vi "EDGE DETECTION REPORT.vi"(8 "error in (no error)":errorcluster, 9 "return value 2":cluster{string, string, dbl, dbl, dbl}, 10 "return value":cluster{string, dbl, dbl, dbl}, 11 "Main Ref":T1) -> (0 "error out":errorcluster)   [LabVIEW 2025]
uses:
  <vilib>/Exaprom PDF/Controls/Font Controls/Font complete cluster.ctl
  <vilib>/Exaprom PDF/Controls/Font Controls/Font size.ctl
  <vilib>/Exaprom PDF/Controls/Font Controls/Font color.ctl
  <vilib>/Exaprom PDF/Controls/Font Controls/Type and encoding.ctl
  <vilib>/Exaprom PDF/Controls/Text Controls/Unicode/Type and run direction.ctl
  <vilib>/Exaprom PDF/Controls/Header, Footer and Watermark Controls/Header or Footer  Text cluster.ctl
  <vilib>/Exaprom PDF/Controls/Table Controls/Cell Alignment 20px.ctl
  <vilib>/Exaprom PDF/Controls/Text Controls/Line spacing.ctl
  <vilib>/Exaprom PDF/Controls/Font Controls/Font complete cluster horizontal.ctl
  <vilib>/Exaprom PDF/Controls/Header, Footer and Watermark Controls/Header or Footer Line cluster.ctl
  <vilib>/Exaprom PDF/Controls/Header, Footer and Watermark Controls/Header Footer Line.ctl
  <vilib>/Exaprom PDF/Controls/Header, Footer and Watermark Controls/Watermark Text Cluster.ctl
  <vilib>/Exaprom PDF/Controls/Header, Footer and Watermark Controls/Watermark Position.ctl
  <vilib>/Exaprom PDF/Controls/Header, Footer and Watermark Controls/Header footer horiz alignment.ctl
  <vilib>/Exaprom PDF/Controls/Table Controls/Table properties.ctl
  <vilib>/Exaprom PDF/Controls/Table Controls/Table position.ctl
  <vilib>/Exaprom PDF/Controls/Header, Footer and Watermark Controls/Header or Footer.ctl
  <vilib>/Exaprom PDF/Controls/Image Controls/Image border.ctl
  <vilib>/Exaprom PDF/Controls/Header, Footer and Watermark Controls/Header or Footer  Image cluster.ctl
  <vilib>/Exaprom PDF/Controls/Table Controls/Cell Font, type, Alignment and LS V2.ctl
  <vilib>/Exaprom PDF/Controls/Table Controls/Cell Type, Alignment and LS.ctl
  <vilib>/Exaprom PDF/Controls/Table Controls/Text vertical arrangement.ctl
  <vilib>/Exaprom PDF/Controls/Image Controls/Image alignment and position.ctl
  <vilib>/Exaprom PDF/Controls/Image Controls/Image aligment.ctl
  <vilib>/Exaprom PDF/VIs/Low level/Header, Footer and Watermark Low level/Append Image HF.vi
  <vilib>/Exaprom PDF/VIs/Low level/Header, Footer and Watermark Low level/Append Text HF.vi
  <vilib>/Exaprom PDF/VIs/Low level/Header, Footer and Watermark Low level/AppendLine seperator.vi
  <vilib>/Exaprom PDF/VIs/Text/Append Phrase.vi
  <vilib>/Exaprom PDF/VIs/Low level/Header, Footer and Watermark Low level/Append Watermark Text.vi
panel:
  in  "Watermark Text 2":T2={"Text "="PALTRO", "Opacity (%)"=5.0, "Position"={"Position"=enum."Center (text section)", "X"=0.0, "Y"=0.0}, "Automatic"=TRUE, "Font"={"Font Name"="", "Size"=-1.0, "Color"=0}, "Alignment"=enum."Center", "Rotate(°)"=0.0}
  in  "Footer Line 2":T7={"H/F Line"=enum."Horizontal line", "Thickness (point)"=0.75, " Colour"=7171459}
  in  "Header Line":T7={"H/F Line"=enum."Horizontal line", "Thickness (point)"=0.75, " Colour"=7171459}
  in  "Footer Text":T9={"Start at page"=1, "Cell Alignment"=4, "Line spacing"=enum."Select", "Text"="Fully automated next-gen fuel and lubricant testers: BOCLE 2.0 , HFRR adv , FBT 3.0", "Font complete"={"Name"="", "Size"=6.0, "Color"=16777224, "Style"={"Bold"=FALSE, "Italic"=FALSE, "Underline"=TRUE, "Strikeout"=FALSE}, "Type"={"Type&direction"=enum."Select", "Embedded"=FALSE, "Encoding"=""}}, "Link"="https://www.paltro.com/products/product-selector/lubricity"}
  in  "Date and Time :":string
  in  "Observations :":string
  in  "Scar Image Path :":path
  in  "Header or footer":T9={"Start at page"=1, "Cell Alignment"=4, "Line spacing"=enum."Select", "Text"="                                            ", "Font complete"={"Name"="", "Size"=-1.0, "Color"=0, "Style"={"Bold"=FALSE, "Italic"=FALSE, "Underline"=FALSE, "Strikeout"=FALSE}, "Type"={"Type&direction"=enum."Select", "Embedded"=FALSE, "Encoding"=""}}, "Link"=""}
  in  "Font":T15={"Name"="", "Size"=18.0, "Color"=0, "Style"={"Bold"=TRUE, "Italic"=FALSE, "Underline"=FALSE, "Strikeout"=FALSE}, "Type"={"Type&direction"=enum."Select", "Embedded"=FALSE, "Encoding"=""}}
  in  "Font 2":T15={"Name"="", "Size"=6.0, "Color"=0, "Style"={"Bold"=FALSE, "Italic"=TRUE, "Underline"=FALSE, "Strikeout"=FALSE}, "Type"={"Type&direction"=enum."Select", "Embedded"=FALSE, "Encoding"=""}}
  in  "File Name :":string(combo)
  out "folder names":string[](array[string])
  out "path out":path
  in  "Automated":bool
  in  "Test Method":string
  in  "Fuel Description":string
  out "Operator :":string
types:
  T1 = cluster{"File Name":string, "Test Method":string, "Operator":string, "Fuel Description":string, "Date and time":string}
  T2 = typedef "Watermark Text Cluster.ctl" = cluster{"Text ":string, "Opacity (%)":sgl, "Position":cluster{"Position":T3, "X":sgl, "Y":sgl}, "Automatic":bool, "Font":cluster{"Font Name":string, "Size":T4, "Color":T5}, "Alignment":T6, "Rotate(°)":sgl}
  T3 = typedef "Watermark Position.ctl" = enum16{"Absolute", "Center (page)", "Center (text section)"}
  T4 = typedef "Font size.ctl" = sgl
  T5 = typedef "Font color.ctl" = u32
  T6 = typedef "Header footer horiz alignment.ctl" = enum16{"Left", "Center", "Right"}
  T7 = typedef "Header or Footer Line cluster.ctl" = cluster{"H/F Line":T8, "Thickness (point)":sgl, " Colour":u32}
  T8 = typedef "Header Footer Line.ctl" = enum16{"No line", "Horizontal line"}
  T9 = typedef "Header or Footer  Text cluster.ctl" = cluster{"Start at page":i32, "Cell Alignment":T10, "Line spacing":T11, "Text":string, "Font complete":T12, "Link":string}
  T10 = typedef "Cell Alignment 20px.ctl" = u16
  T11 = typedef "Line spacing.ctl" = enum16{"Select", "1.0", "1.5", "2.0"}
  T12 = typedef "Font complete cluster horizontal.ctl" = cluster{"Name":string, "Size":T4, "Color":T5, "Style":cluster{"Bold":bool, "Italic":bool, "Underline":bool, "Strikeout":bool}, "Type":T13}
  T13 = typedef "Type and encoding.ctl" = cluster{"Type&direction":T14, "Embedded":bool, "Encoding":string}
  T14 = typedef "Type and run direction.ctl" = enum16{"Select", "ASCII", "UTF-16", "UTF-16 (default)", "UTF-16 (LTR)", "UTF-16 (RTL)"}
  T15 = typedef "Font complete cluster.ctl" = cluster{"Name":string, "Size":T4, "Color":T5, "Style":cluster{"Bold":bool, "Italic":bool, "Underline":bool, "Strikeout":bool}, "Type":T13}
  T16 = typedef "Image alignment and position.ctl" = cluster{"Alignment":T17, "X ":sgl, "Y":sgl, "Indentation":sgl}
  T17 = typedef "Image aligment.ctl" = enum16{"Absolute (X,Y)", "Left", "Center", "Right", "Left (textwrap)", "Right (textwrap)"}
  T18 = typedef "Image border.ctl" = cluster{"Show?":bool, "Thickness (point)":sgl, "Color":u32}
  T19 = typedef "Cell Font, type, Alignment and LS V2.ctl" = cluster{"Cell Type, Alignment and LS":T20, "Font":T15}
  T20 = typedef "Cell Type, Alignment and LS.ctl" = cluster{"Cell Alignment":T10, "Text rotation":T21, "Line spacing":T11}
  T21 = typedef "Text vertical arrangement.ctl" = enum16{"None", "Clockwise", "Counterclockwise"}
  T22 = typedef "Header or Footer  Image cluster.ctl" = cluster{"Start at page":i32, "Cell Alignment":T10, "Path":path, "Image (%)":sgl, "Link":string}
  T23 = typedef "Table properties.ctl" = cluster{"Table position":T24, "SpacingBefore (points)":sgl, "SpacingAfter (points)":sgl}
  T24 = typedef "Table position.ctl" = i32
  T25 = typedef "Header or Footer.ctl" = enum16{"Header", "Footer"}
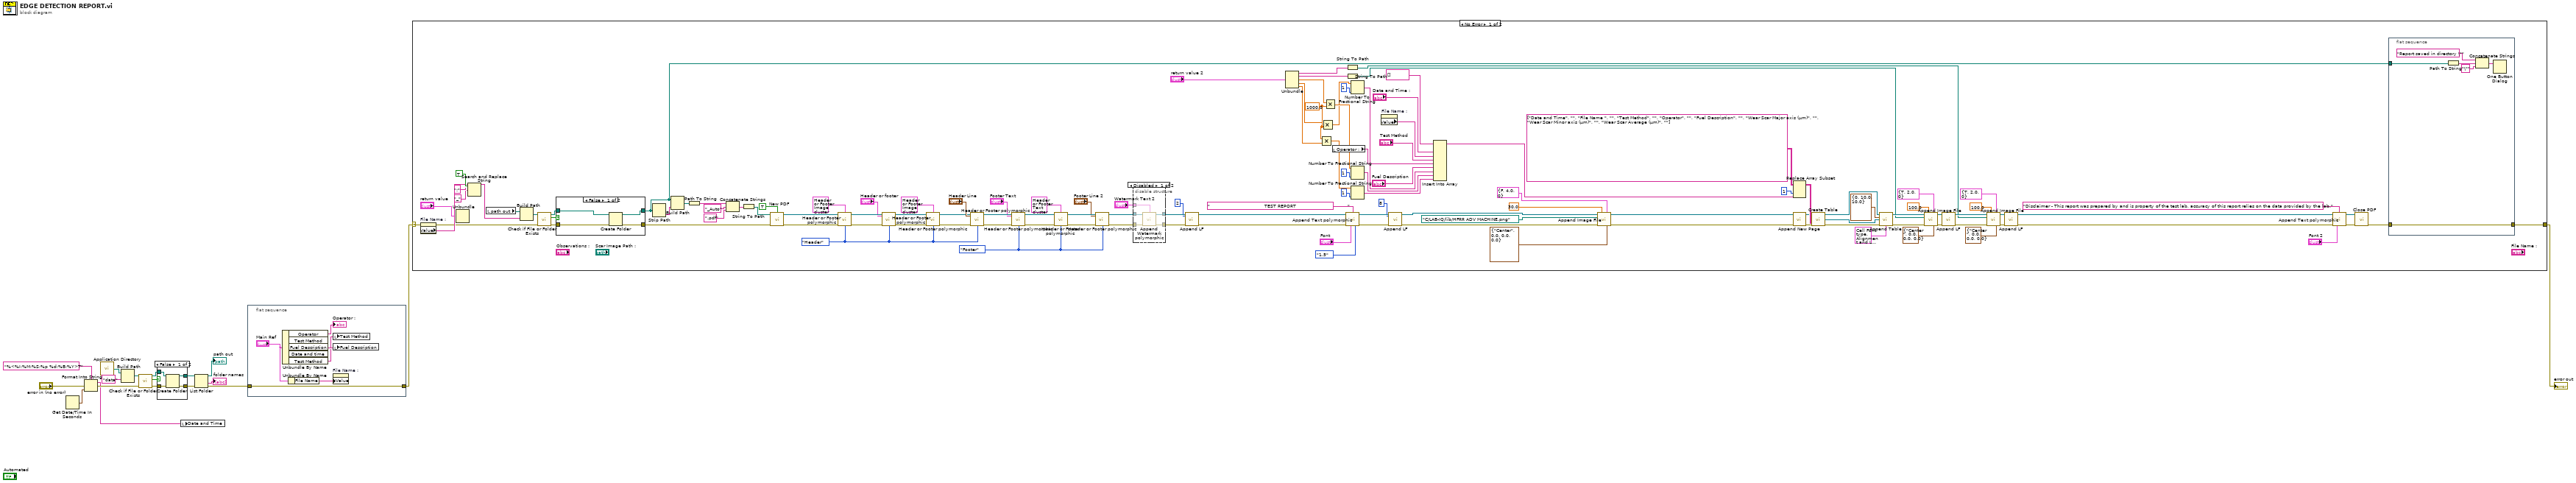
[diagram p0: block diagram]
diagram:
  n1 = Get Date/Time In Seconds() -> (seconds since 1Jan1904=w7:timestamp)
  n2 = Format Into String(format string="%<%I:%M:%S:%p %d:%B:%Y>T", error in="error in (no error)", w7) -> (resulting string=w1:string, error out=w5:errorcluster)  [unwired: 1 in]
  n3 = call <vilib>:"Application Directory.vi"() -> ("Application Directory"=w9:path)
  n4 = Build Path(base path=w9, name or relative path="data") -> (appended path=w8:path)
  n5 = call <vilib>:"Check if File or Folder Exists.vi"("error in (no error)"=w5, "path"=w8) -> ("error out"=w13:errorcluster, "file or folder exists?"=w15:bool, "dup path"=w14:path)  [unwired: 7 in]
  n6 = case shown="False" w15 {
    tunnel: w14 -> [w22 w23]
    tunnel: w13 -> [w21 w24]
    tunnel: [w20 w24] -> w18
    tunnel: [w19 w23] -> w16
    frame False {
      n7 = Create Folder(path (use dialog)=w22, error in=w21) -> (created path=w19:path, error out=w20:errorcluster)  [unwired: 1 in, 1 out]
    }
    frame True {
    }
  }
  n8 = local write "Date and Time :"(w1) -> ()
  n9 = List Folder(path=w16, error in=w18) -> (path out=→"path out":path, folder names=→"folder names":string[], error out=w3:errorcluster)  [unwired: 2 in, 1 out]
  n10 = flat-sequence {
    tunnel: w3 -> [w26]
    tunnel: [w26] -> w2
    frame #0 {
      n11 = Unbundle By Name("Main Ref") -> ("Operator"=→"Operator :":string, "Fuel Description"=w27:string, "Test Method"=w25:string)  [unwired: 2 out]
      n12 = Unbundle By Name("Main Ref") -> ("File Name"=w30:string)
      n13 = local write "Test Method"(w25) -> ()
      n14 = local write "Fuel Description"(w27) -> ()
      n15 = property on="File Name :" class="CmbBox"("Value"=w30) -> ()  [unwired: 2 in, 2 out]
    }
  }
  n16 = case shown="No Error" w2 {
    selector: w2 -> [w64 _]
    tunnel: [w59 _] -> w11
    frame No Error {
      w38 = 1000.0 ("y")
      w79 = Header_or_Footer."Header" ("Position")
      w109 = Header_or_Footer."Footer" ("Position")
      n17 = property on="File Name :" class="CmbBox"(error in=w64) -> (error out=w68:errorcluster, "Value"=w69:string)  [unwired: 1 in, 1 out]
      n18 = Unbundle("return value") -> ()  [unwired: 4 out]
      n19 = Search and Replace String(replace all?=TRUE ("replace all? (F)"), input string=w69, search string=":", replace string="_" ("replace string (\"\")")) -> (result string=w99:string)  [unwired: 4 in, 3 out]
      n20 = local read "path out"() -> (w70:path)
      n21 = Build Path(base path=w70, name or relative path=w99) -> (appended path=w126:path)
      n22 = call <vilib>:"Check if File or Folder Exists.vi"("error in (no error)"=w68, "path"=w126) -> ("error out"=w123:errorcluster, "file or folder exists?"=w125:bool, "dup path"=w124:path)  [unwired: 7 in]
      n23 = case shown="False" w125 {
        tunnel: w124 -> [w172 w173]
        tunnel: w123 -> [w171 w174]
        tunnel: [w170 w174] -> w122
        tunnel: [w169 w173] -> w71
        frame False {
          n24 = Create Folder(path (use dialog)=w172, error in=w171) -> (created path=w169:path, error out=w170:errorcluster)  [unwired: 1 in, 1 out]
        }
        frame True {
        }
      }
      n25 = Strip Path(path=w71) -> (name=w128:string)  [unwired: 1 out]
      n26 = Build Path(base path=w71, name or relative path=w128) -> (appended path=w127:path)
      n27 = Path To String(path=w127) -> (string=w58:string)
      n28 = Concatenate Strings(w58, "_Auto" ("string"), ".pdf" ("string")) -> (w129:string)
      n29 = String To Path(string=w129) -> (path=w121:path)
      n30 = call <vilib>:"New PDF.vi"("PDF Path"=w121, "Overwrite?"=TRUE, "error in (no error)"=w122) -> ("PDF Report"=w143:refnum<class "PDF Report Class.lvclass">, "error out"=w144:errorcluster)  [unwired: 11 in]
      n31 = call-poly <vilib>:"Header or Footer polymorphic.vi"("PDF Report IN"=w143, "Header or footer"=T22 {"Start at page"=1, "Cell Alignment"=4, "Path"=path "C:/LAB-IQ/lib/paltro logo.png", "Image (%)"=100.0, "Link"="https://www.paltro.com/"} ("HEADER Image"), "error in (no error)"=w144, "Position"=w79) -> ("PDF Report OUT"=w97:refnum<class "PDF Report Class.lvclass">, "error out"=w98:errorcluster)  [unwired: 10 out]
      n32 = call-poly <vilib>:"Header or Footer polymorphic.vi"("PDF Report IN"=w97, "Header or footer"="Header or footer", "error in (no error)"=w98, "Position"=w79) -> ("PDF Report OUT"=w95:refnum<class "PDF Report Class.lvclass">, "error out"=w96:errorcluster)  [unwired: 10 out]
      n33 = call-poly <vilib>:"Header or Footer polymorphic.vi"("PDF Report IN"=w95, "Header or footer"=T22 {"Start at page"=1, "Cell Alignment"=6, "Path"=path "C:/LAB-IQ/lib/HFRR_adv.png", "Image (%)"=30.0, "Link"="https://www.paltro.com/products/test-and-measurement/bocle--automated-ball-on-cylinder-lubricity-evaluator"} ("HEADER Image  2"), "error in (no error)"=w96, "Position"=w79) -> ("PDF Report OUT"=w115:refnum<class "PDF Report Class.lvclass">, "error out"=w116:errorcluster)  [unwired: 10 out]
      n34 = call-poly <vilib>:"Header or Footer polymorphic.vi"("PDF Report IN"=w115, "H/F Line"="Header Line", "error in (no error)"=w116, "Position"=w79) -> ("PDF Report OUT"=w147:refnum<class "PDF Report Class.lvclass">, "error out"=w146:errorcluster)  [unwired: 1 in, 9 out]
      n35 = call-poly <vilib>:"Header or Footer polymorphic.vi"("PDF Report IN"=w147, "Header or footer"="Footer Text", "error in (no error)"=w146, "Position"=w109) -> ("PDF Report OUT"=w149:refnum<class "PDF Report Class.lvclass">, "error out"=w148:errorcluster)  [unwired: 10 out]
      n36 = call-poly <vilib>:"Header or Footer polymorphic.vi"("PDF Report IN"=w149, "Header or footer"=T9 {"Start at page"=1, "Cell Alignment"=6, "Line spacing"=enum."Select", "Text"="www.paltro.com", "Font complete"={"Name"="", "Size"=6.0, "Color"=16777224, "Style"={"Bold"=FALSE, "Italic"=FALSE, "Underline"=TRUE, "Strikeout"=FALSE}, "Type"={"Type&direction"=enum."Select", "Embedded"=FALSE, "Encoding"=""}}, "Link"="https://www.paltro.com/"} ("Footer Text 2"), "error in (no error)"=w148, "Position"=w109) -> ("PDF Report OUT"=w142:refnum<class "PDF Report Class.lvclass">, "error out"=w141:errorcluster)  [unwired: 10 out]
      n37 = call-poly <vilib>:"Header or Footer polymorphic.vi"("PDF Report IN"=w142, "H/F Line"="Footer Line 2", "error in (no error)"=w141, "Position"=w109) -> ("PDF Report OUT"=w135:refnum<class "PDF Report Class.lvclass">, "error out"=w136:errorcluster)  [unwired: 1 in, 9 out]
      n38 = disable-structure shown="Disabled" {
        disable-tunnel: "Watermark Text 2" -> [w166 _]
        disable-tunnel: w136 -> [w165 w168]
        disable-tunnel: w135 -> [w164 w167]
        disable-tunnel: [w163 w168] -> w91
        disable-tunnel: [w162 w167] -> w90
        frame Disabled {
          n39 = call-poly <vilib>:"Append Watermark polymorphic.vi"("PDF Report IN"=w164, "Watermark Text"=w166, "error in (no error)"=w165) -> ("PDF Report OUT"=w162:refnum<class "PDF Report Class.lvclass">, "error out"=w163:errorcluster)  [unwired: 1 in, 10 out]
        }
        frame Enabled {
        }
      }
      n40 = call <vilib>:"Append LF.vi"("PDF Report IN"=w90, "Number of LF (default 1)"=u8 2, "error in (no error)"=w91) -> ("PDF Report duplicate"=w88:refnum<class "PDF Report Class.lvclass">, "error out"=w89:errorcluster)  [unwired: 11 in]
      n41 = Unbundle("return value 2") -> (w44:string, w45:string, w37:dbl, w36:dbl, w35:dbl)
      n42 = Multiply(x=w38, y=w35) -> (x*y=w32:dbl)
      n43 = Multiply(x=w36, y=w38) -> (x*y=w33:dbl)
      n44 = Multiply(x=w37, y=w38) -> (x*y=w34:dbl)
      n45 = local read "Operator :"() -> (w31:string)
      n46 = String To Path(string=w44) -> (path=w42:path)
      n47 = String To Path(string=w45) -> (path=w43:path)
      n48 = call-poly <vilib>:"Append Text polymorphic.vi"("PDF Report IN"=w88, "Text"="                                     TEST REPORT                                   ", "error in (no error)"=w89, "Font"="Font", "Line spacing"=Line_spacing."1.5") -> ("PDF Report OUT"=w75:refnum<class "PDF Report Class.lvclass">, "error out"=w76:errorcluster)  [unwired: 9 in]
      n49 = Number To Fractional String(number=w33, precision (6)=i16 1) -> (F-format string=w39:string)  [unwired: 2 in]
      n50 = Number To Fractional String(number=w34, precision (6)=i16 1) -> (F-format string=w40:string)  [unwired: 2 in]
      n51 = Number To Fractional String(number=w32, precision (6)=i16 1) -> (F-format string=w41:string)  [unwired: 2 in]
      n52 = property on="File Name :" class="CmbBox"() -> ("Value"=w67:string)  [unwired: 2 in, 2 out]
      n53 = call <vilib>:"Append LF.vi"("PDF Report IN"=w75, "Number of LF (default 1)"=u8 8, "error in (no error)"=w76) -> ("PDF Report duplicate"=w78:refnum<class "PDF Report Class.lvclass">, "error out"=w77:errorcluster)  [unwired: 11 in]
      n54 = Insert Into Array(array=string[] [], new element #1="Date and Time :", new element #2=w67, new element #3="Test Method", new element #4=w31, new element #5="Fuel Description", new element #6=w39, new element #7=w40, new element #8=w41) -> (w151:string[])  [unwired: 1 in]
      n55 = call <vilib>:"Append Image File.vi"("PDF Report IN"=w78, "Scale (%)"=sgl 30.0, "Border"=T18 {"Show?"=FALSE, "Thickness (point)"=4.0, "Color"=0}, "Image path"=path "C:/LAB-IQ/lib/HFRR ADV MACHINE.png", "error in (no error)"=w77, "Position and indentation"=T16 {"Alignment"=enum."Center", "X "=0.0, "Y"=0.0, "Indentation"=0.0}) -> ("PDF Report OUT"=w119:refnum<class "PDF Report Class.lvclass">, "error out"=w120:errorcluster)  [unwired: 6 in, 2 out]
      n56 = Replace Array Subset(array=string[][] [["Date and Time", ""], ["File Name ", ""], ["Test Method", ""], ["Operator", ""], ["Fuel Description", ""], ["Wear Scar Major axis (µm)", ""], ["Wear Scar Minor axis (µm)", ""], ["Wear Scar Average (µm)", ""]] ("Text Data 2D [ ]"), new element=w151, index (col)=1 ("disabled index (col)")) -> (w152:string[][])  [unwired: 1 in]
      n57 = call <vilib>:"Append New Page.vi"("PDF Report"=w119, "error in (no error)"=w120) -> ("PDF Report duplicate"=w117:refnum<class "PDF Report Class.lvclass">, "error OUT"=w118:errorcluster)  [unwired: 12 in]
      n58 = call <vilib>:"Create Table.vi"("PDF Report IN"=w117, "Text Data 2D [ ]"=w152, "error in (no error)"=w118) -> ("PDF Report duplicate"=w132:refnum<class "PDF Report Class.lvclass">, "PDF Table"=w134:refnum<class "Pdfp Table Class.lvclass">, "error out"=w130:errorcluster)  [unwired: 10 in]
      n59 = call <vilib>:"Append Table.vi"("PDF Report IN"=w132, "Table properties"=T23 {"Table position"=0, "SpacingBefore (points)"=10.0, "SpacingAfter (points)"=10.0} ("Table properties  - Tables 2 to 4"), "PDF Table"=w134, "error in (no error)"=w130, "Datas format"=T19 {"Cell Type, Alignment and LS"={"Cell Alignment"=4, "Text rotation"=enum."None", "Line spacing"=enum."Select"}, "Font"={"Name"="", "Size"=-1.0, "Color"=0, "Style"={"Bold"=FALSE, "Italic"=FALSE, "Underline"=FALSE, "Strikeout"=FALSE}, "Type"={"Type&direction"=enum."Select", "Embedded"=FALSE, "Encoding"=""}}}) -> ("PDF Report OUT"=w133:refnum<class "PDF Report Class.lvclass">, "error out"=w131:errorcluster)  [unwired: 7 in, 2 out]
      n60 = call <vilib>:"Append Image File.vi"("PDF Report IN"=w133, "Scale (%)"=sgl 100.0, "Border"=T18 {"Show?"=TRUE, "Thickness (point)"=2.0, "Color"=0}, "Image path"=w43, "error in (no error)"=w131, "Position and indentation"=T16 {"Alignment"=enum."Center", "X "=0.0, "Y"=0.0, "Indentation"=0.0}) -> ("PDF Report OUT"=w81:refnum<class "PDF Report Class.lvclass">, "error out"=w82:errorcluster)  [unwired: 6 in, 2 out]
      n61 = call <vilib>:"Append LF.vi"("PDF Report IN"=w81, "error in (no error)"=w82) -> ("PDF Report duplicate"=w49:refnum<class "PDF Report Class.lvclass">, "error out"=w50:errorcluster)  [unwired: 12 in]
      n62 = call <vilib>:"Append Image File.vi"("PDF Report IN"=w49, "Scale (%)"=sgl 100.0, "Border"=T18 {"Show?"=TRUE, "Thickness (point)"=2.0, "Color"=0}, "Image path"=w42, "error in (no error)"=w50, "Position and indentation"=T16 {"Alignment"=enum."Center", "X "=0.0, "Y"=0.0, "Indentation"=0.0}) -> ("PDF Report OUT"=w54:refnum<class "PDF Report Class.lvclass">, "error out"=w53:errorcluster)  [unwired: 6 in, 2 out]
      n63 = call <vilib>:"Append LF.vi"("PDF Report IN"=w54, "error in (no error)"=w53) -> ("PDF Report duplicate"=w46:refnum<class "PDF Report Class.lvclass">, "error out"=w47:errorcluster)  [unwired: 12 in]
      n64 = call-poly <vilib>:"Append Text polymorphic.vi"("PDF Report IN"=w46, "Text"="Disclaimer - This report was prepared by and is property of the test lab, accuracy of this report relies on the data provided by the lab.", "error in (no error)"=w47, "Font"="Font 2") -> ("PDF Report OUT"=w84:refnum<class "PDF Report Class.lvclass">, "error out"=w85:errorcluster)  [unwired: 10 in]
      n65 = call <vilib>:"Close PDF.vi"("PDF Report"=w84, "error in (no error)"=w85) -> ("error out"=w72:errorcluster)  [unwired: 12 in, 1 out]
      n66 = flat-sequence {
        tunnel: w72 -> [w161]
        tunnel: [w161] -> w59
        tunnel: w71 -> [w160]
        frame #0 {
          n67 = Path To String(path=w160) -> (string=w159:string)
          n68 = Concatenate Strings("Report saved in directory \"", w159, "\"" ("string")) -> (w156:string)
          n69 = One Button Dialog(message=w156) -> ()  [unwired: 1 in, 1 out]
        }
      }
    }
    frame Error {
      # "WHEN USER PRESSED CLOSE BUTTON"
    }
  }
  "error out" <- w11
